vi "IT6333A_Set Resource Name.vi"(8 "error in (no error)":errorcluster, 10 "Resource Name":string, 11 "PowerSupply_IT6333A in":refnum<class "PowerSupply_IT6333A.lvclass">) -> (0 "error out":errorcluster, 3 "PowerSupply_IT6333A out":refnum<class "PowerSupply_IT6333A.lvclass">)   [LabVIEW 2017, in "PowerSupply_IT6333A.lvclass"]
uses:
  PowerSupply_IT6333A.lvclass
  PowerSupply_IT6333A.lvclass/PowerSupply_IT6333A.ctl
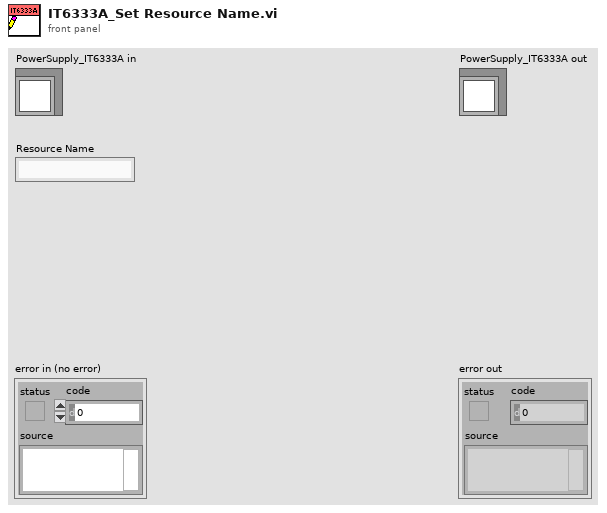
[diagram p1: front panel]
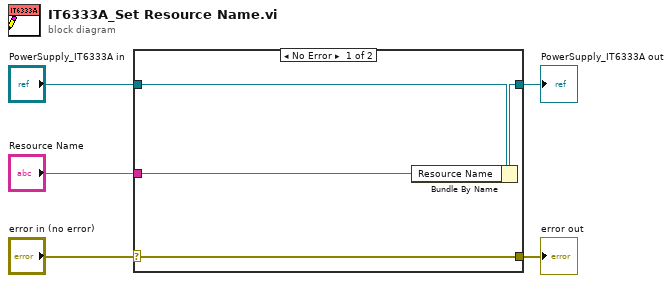
[diagram p0: block diagram]
diagram:
  n1 = case shown="No Error" "error in (no error)" {
    selector: "error in (no error)" -> [w9 w10]
    tunnel: [w9 w10] -> w4
    tunnel: [w7 w11] -> w2
    tunnel: "PowerSupply_IT6333A in" -> [w8 w11]
    tunnel: "Resource Name" -> [w6 _]
    frame No Error {
      n2 = Bundle By Name(cluster=w8, "Resource Name"=w6) -> (w7:refnum<class "PowerSupply_IT6333A.lvclass">)
    }
    frame Error {
    }
  }
  "error out" <- w4
  "PowerSupply_IT6333A out" <- w2
